vi "DSF.Engine.Memory.ObjectPool.Obtain Index.vi"(8 "error in (no error)":errorcluster, 9 "timeout ms (0)":i32 format="%d ms", 11 "ObjectPool in":refnum<class "DSF.Engine.Memory.ObjectPool.lvclass">) -> (0 "error out":errorcluster, 1 "timed out?":bool, 2 "index":i32, 3 "ObjectPool out":refnum<class "DSF.Engine.Memory.ObjectPool.lvclass">)   [LabVIEW 2016, in "DSF.Engine.lvlib" / "DSF.Engine.Memory.ObjectPool.lvclass"]
uses:
  DSF.Engine.Memory.ObjectPool.lvclass
  DSF.Engine.Memory.ObjectPool.lvclass/DSF.Engine.Memory.ObjectPool.ctl
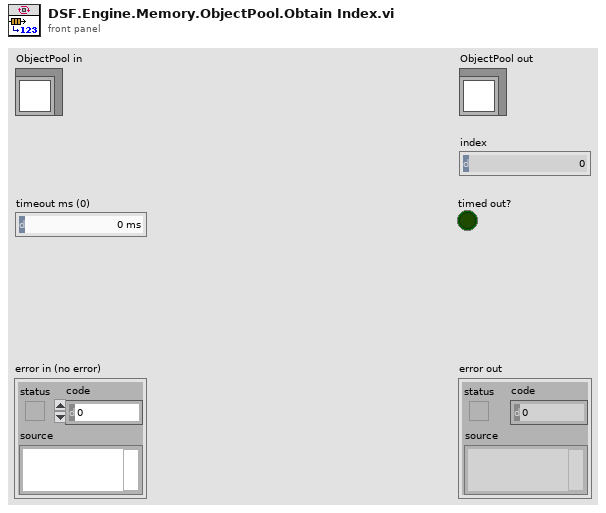
[diagram p1: front panel]
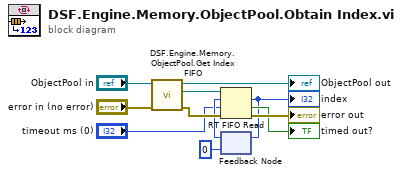
[diagram p0: block diagram]
diagram:
  n1 = call "DSF.Engine.Memory.ObjectPool.Get Index FIFO.vi"("error in (no error)"="error in (no error)", "ObjectPool in"="ObjectPool in") -> ("error out"=w5:errorcluster, "Index FIFO"=w11:refnum<k33>, "ObjectPool out"=→"ObjectPool out":refnum<class "DSF.Engine.Memory.ObjectPool.lvclass">)  [unwired: 7 in]
  n2 = feedback #1(0) -> (w2:i32)
  n3 = RT FIFO Read(0:w11, 1:w2, 2:"timeout ms (0)", 3:w5) -> (9:w3:i32, 10:→"timed out?":bool, 11:→"error out":errorcluster)  [unwired: 2 out]
  "index" <- w3
  n4 = feedback-in #1(w3) -> ()
